vi "JoyScaleTank.vi"(8 "Tolerance":dbl, 10 "x Axis":dbl(slide) scale=-127.0..127.0, 11 "y Axis":dbl(slide) scale=-127.0..127.0 scale format="%#_4g") -> (1 "Speed Right":dbl(knob) scale=-1.0..1.0, 2 "Speed Left":dbl(knob) scale=-1.0..1.0, 3 "Speed":dbl(knob) scale=-1.0..1.0)   [LabVIEW 2011]
panel:
  out "Pos Tolerance":dbl
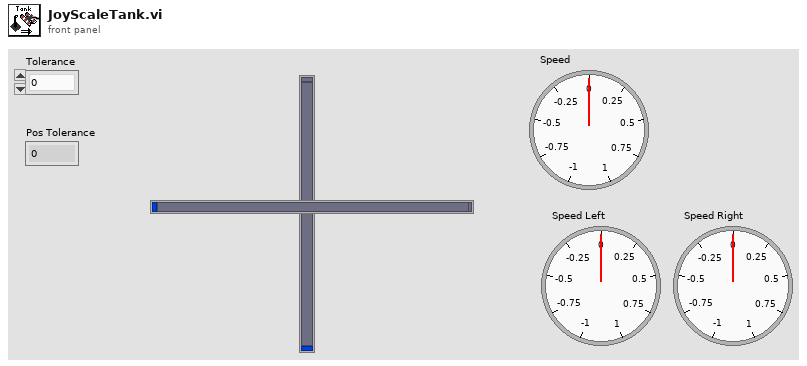
[diagram p1: front panel]
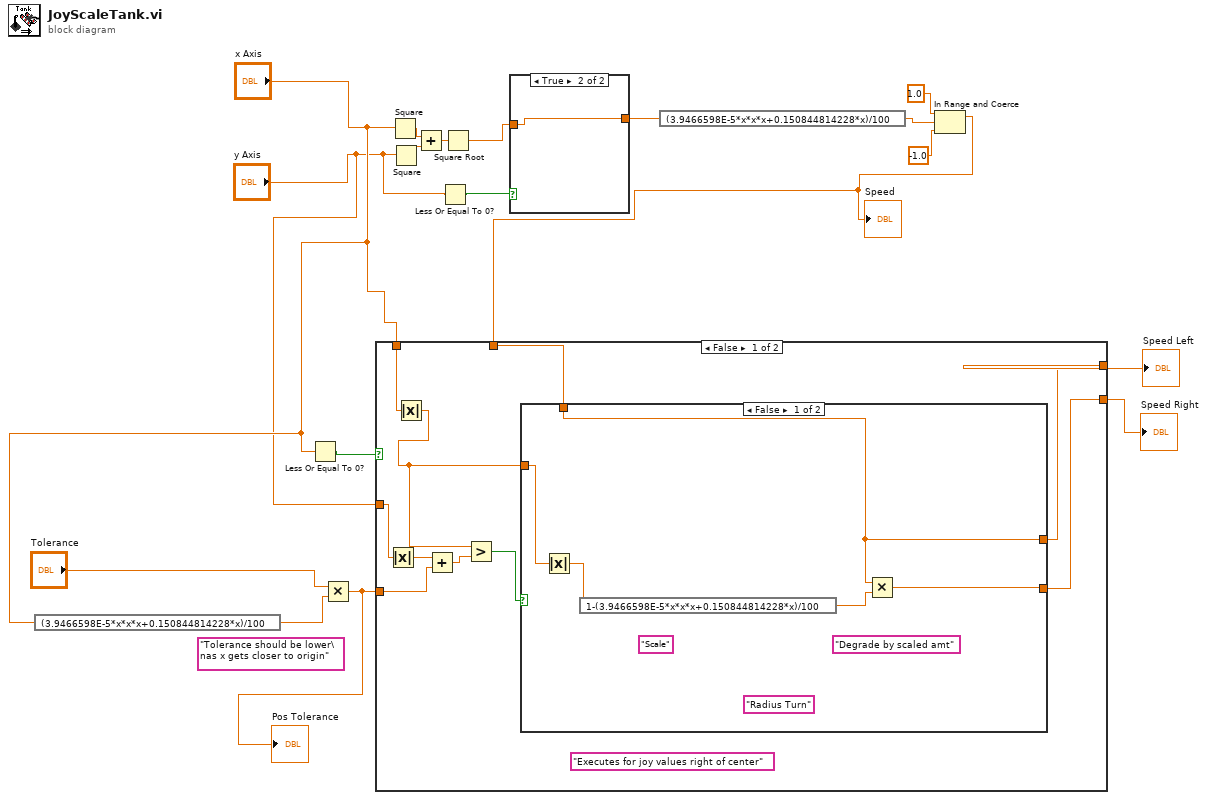
[diagram p0: block diagram]
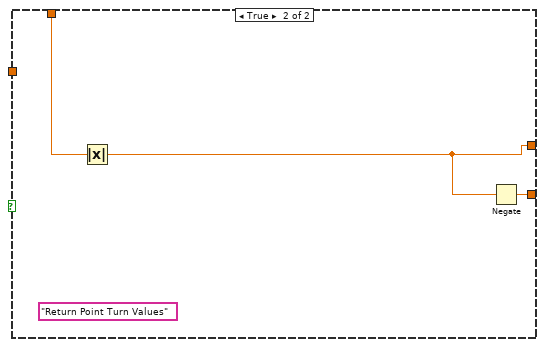
[diagram p2: hidden frame]
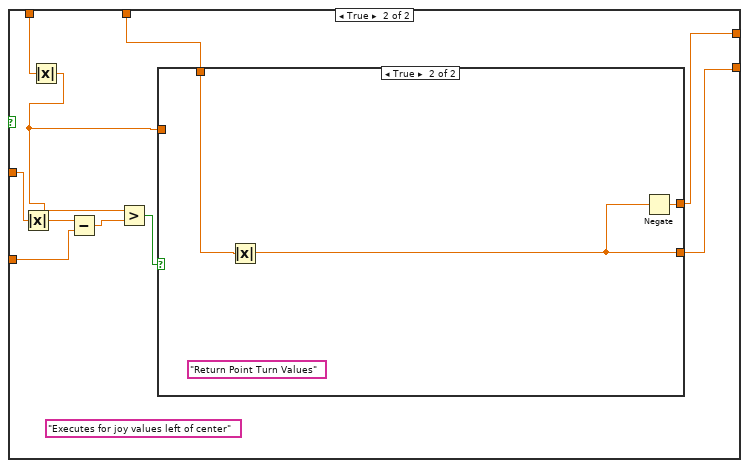
[diagram p3: hidden frame]
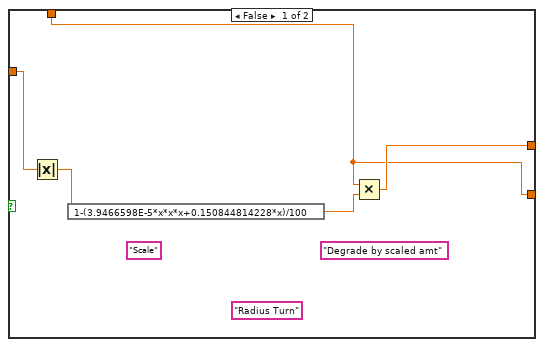
[diagram p4: hidden frame]
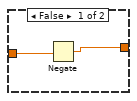
[diagram p5: hidden frame]
diagram:
  (unwired) "Tolerance should be lower\nas x gets closer to origin"
  n1 = expression code="(3.9466598E-5*x*x*x+0.150844814228*x)/100"("x Axis") -> (w6:dbl)
  n2 = Less Or Equal To 0?(x="x Axis") -> (x <= 0?=w11:bool)
  n3 = Multiply(x="Tolerance", y=w6) -> (x*y=w4:dbl)
  "Pos Tolerance" <- w4
  n4 = Square(x="x Axis") -> (x^2=w16:dbl)
  n5 = Square(x="y Axis") -> (x^2=w17:dbl)
  n6 = Add(x=w16, y=w17) -> (x+y=w18:dbl)
  n7 = Less Or Equal To 0?(x="y Axis") -> (x <= 0?=w1:bool)
  n8 = Square Root(x=w18) -> (sqrt(x)=w14:dbl)
  n9 = case shown="True" w1 {
    tunnel: [w19 w21] -> w15
    tunnel: w14 -> [w20 w21]
    frame False {
      n10 = Negate(x=w20) -> (-x=w19:dbl)
    }
    frame True {
    }
  }
  n11 = expression code="(3.9466598E-5*x*x*x+0.150844814228*x)/100"(w15) -> (w10:dbl)
  n12 = In Range and Coerce(upper limit=1.0, x=w10, lower limit=-1.0) -> (coerced(x)=w7:dbl)  [unwired: 1 out]
  "Speed" <- w7
  n13 = case shown="False" w11 {
    tunnel: [w25 w48] -> w13
    tunnel: "x Axis" -> [w29 w45]
    tunnel: w7 -> [w30 w46]
    tunnel: [w26 w47] -> w12
    tunnel: "y Axis" -> [w27 w43]
    tunnel: w4 -> [w22 w40]
    frame False {
      (unwired) "Executes for joy values right of center"
      n14 = Absolute Value(x=w27) -> (abs(x)=w24:dbl)
      n15 = Absolute Value(x=w29) -> (abs(x)=w28:dbl)
      n16 = Add(x=w24, y=w22) -> (x+y=w23:dbl)
      n17 = Greater?(x=w28, y=w23) -> (0:w31:bool)
      n18 = case shown="False" w31 {
        tunnel: [w33 w38] -> w25
        tunnel: [w32 w37] -> w26
        tunnel: w30 -> [w32 w39]
        tunnel: w28 -> [w34 _]
        frame False {
          (unwired) "Radius Turn"
          (unwired) "Degrade by scaled amt"
          (unwired) "Scale"
          n19 = Absolute Value(x=w34) -> (abs(x)=w35:dbl)
          n20 = expression code="1-(3.9466598E-5*x*x*x+0.150844814228*x)/100"(w35) -> (w36:dbl)
          n21 = Multiply(x=w32, y=w36) -> (x*y=w33:dbl)
        }
        frame True {
          (unwired) "Return Point Turn Values"
          n22 = Absolute Value(x=w39) -> (abs(x)=w37:dbl)
          n23 = Negate(x=w37) -> (-x=w38:dbl)
        }
      }
    }
    frame True {
      (unwired) "Executes for joy values left of center"
      n24 = Absolute Value(x=w43) -> (abs(x)=w41:dbl)
      n25 = Absolute Value(x=w45) -> (abs(x)=w44:dbl)
      n26 = Subtract(x=w41, y=w40) -> (x-y=w42:dbl)
      n27 = Greater?(x=w44, y=w42) -> (0:w49:bool)
      n28 = case shown="True" w49 {
        tunnel: [w50 w55] -> w48
        tunnel: [w51 w57] -> w47
        tunnel: w46 -> [w50 w56]
        tunnel: w44 -> [w52 _]
        frame False {
          (unwired) "Radius Turn"
          (unwired) "Degrade by scaled amt"
          (unwired) "Scale"
          n29 = Absolute Value(x=w52) -> (abs(x)=w53:dbl)
          n30 = expression code="1-(3.9466598E-5*x*x*x+0.150844814228*x)/100"(w53) -> (w54:dbl)
          n31 = Multiply(x=w50, y=w54) -> (x*y=w51:dbl)
        }
        frame True {
          (unwired) "Return Point Turn Values"
          n32 = Absolute Value(x=w56) -> (abs(x)=w55:dbl)
          n33 = Negate(x=w55) -> (-x=w57:dbl)
        }
      }
    }
  }
  "Speed Left" <- w12
  "Speed Right" <- w13
